vi "CRYRecall Curves Select.vi"(0 "Curve Names":string[](array[string]), 5 "Curves Selected?":bool[](array[boolean]), 7 "Row":u32) -> (3 "Table Control":string[][](table), 4 "Sel_1":bool, 6 "Sel_2":bool, 8 "Sel_3":bool, 10 "Sel_4":bool, 14 "Sel_6":bool, 15 "Sel_5":bool)   [LabVIEW 2013]
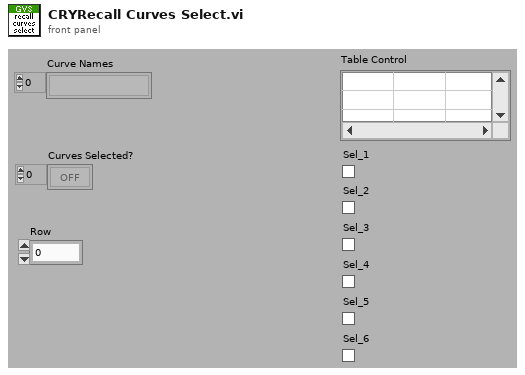
[diagram p1: front panel]
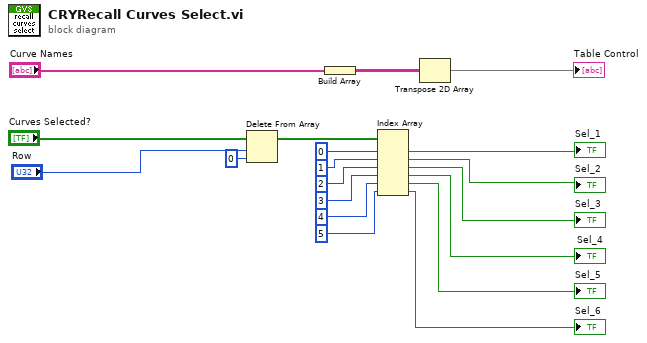
[diagram p0: block diagram]
diagram:
  n1 = Delete From Array(array="Curves Selected?", length="Row", index=0) -> (array with subset deleted=w2:bool[])  [unwired: 1 out]
  n2 = Build Array("Curve Names") -> (w1:string[][])
  n3 = Index Array(array=w2, index #1=0 ("index"), index #2=1 ("index"), index #3=2 ("index"), index #4=3 ("index"), index #5=4 ("index"), index #6=5 ("index")) -> (element #1=→"Sel_1":bool, element #2=→"Sel_2":bool, element #3=→"Sel_3":bool, element #4=→"Sel_4":bool, element #5=→"Sel_5":bool, element #6=→"Sel_6":bool)
  n4 = Transpose 2D Array(2D array=w1) -> (transposed array=→"Table Control":string[][])
